vi "EventLogic.vi"(1 "Recognising":bool, 2 "Processing":bool, 3 "Aborted":bool) -> (0 "WhatToDo":string)   [LabVIEW 2020]
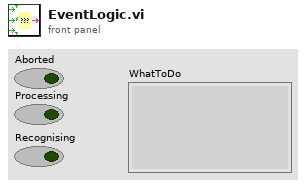
[diagram p1: front panel]
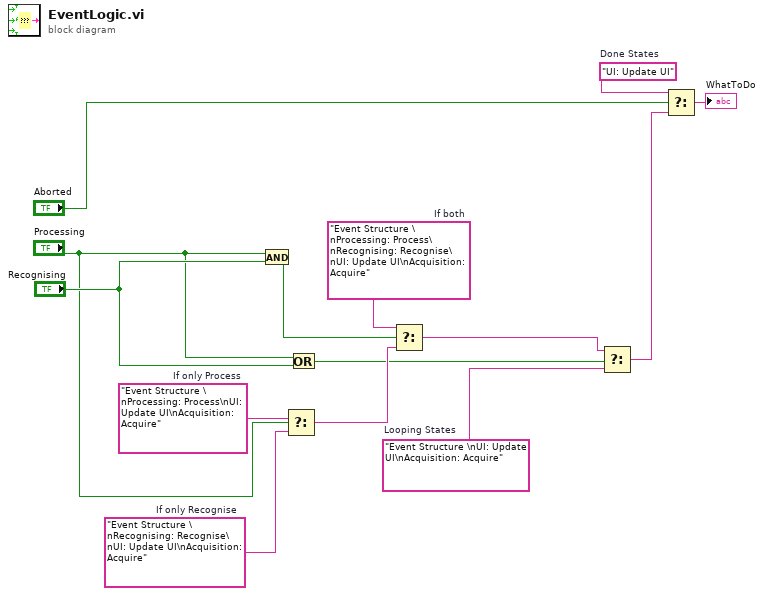
[diagram p0: block diagram]
diagram:
  w6 = "Event Structure \nUI: Update UI\nAcquisition: Acquire"  # Looping States
  w9 = "Event Structure \nRecognising: Recognise\nUI: Update UI\nAcquisition: Acquire"  # If only Recognise
  w10 = "Event Structure \nProcessing: Process\nUI: Update UI\nAcquisition: Acquire"  # If only Process
  w12 = "Event Structure \nProcessing: Process\nRecognising: Recognise\nUI: Update UI\nAcquisition: Acquire"  # If both
  w14 = "UI: Update UI"  # Done States
  n1 = And(x="Processing", y="Recognising") -> (x .and. y?=w13:bool)
  n2 = Select(t=w10, s="Processing", f=w9) -> (s? t:f=w11:string)
  n3 = Or(x="Processing", y="Recognising") -> (x .or. y?=w8:bool)
  n4 = Select(t=w12, s=w13, f=w11) -> (s? t:f=w7:string)
  n5 = Select(t=w7, s=w8, f=w6) -> (s? t:f=w5:string)
  n6 = Select(t=w14, s="Aborted", f=w5) -> (s? t:f=→"WhatToDo":string)
